vi "Curve Length Preparation.vi"(2 "formula":string) -> (0 "correct number of variables":bool, 1 "valid formula":bool, 3 "error":bool, 4 "string without spaces":string, 5 "epsilon with brackets":string, 6 "epsilon without brackets":string, 7 "formula with brackets":string)   [LabVIEW 2020, in "NI_Gmath.lvlib"]
uses:
  NI_Gmath.lvlib
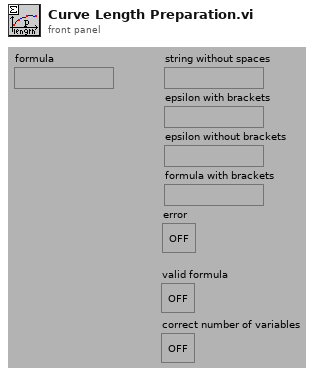
[diagram p1: front panel]
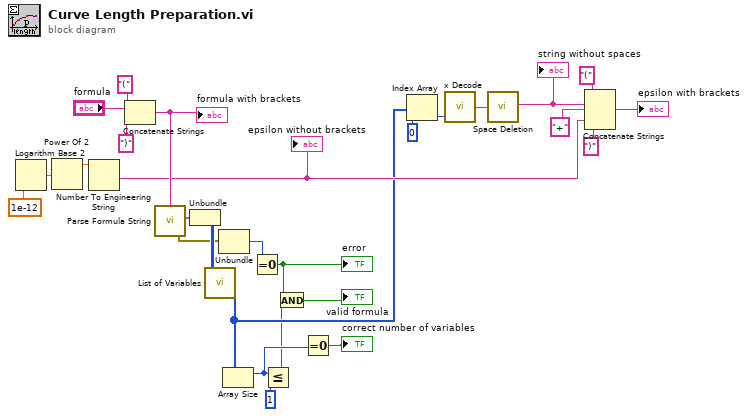
[diagram p0: block diagram]
diagram:
  n1 = Logarithm Base 2(1:1e-12) -> (0:w5:dbl)
  n2 = Power Of 2(x=w5) -> (2^x=w9:dbl)
  n3 = Number To Engineering String(4:w9) -> (0:w14:string)  [unwired: 3 in]
  "epsilon without brackets" <- w14
  n4 = Concatenate Strings("(", "formula", ")") -> (w27:string)
  "formula with brackets" <- w27
  n5 = call "Parse Formula String.vi"("formula"=w27) -> ("error out"=w15:errorcluster, "Parsed Formula"=w20:cluster{"Table":i32[][], "Y Values":dbl[]})  [unwired: 1 in]
  n6 = Unbundle(w20) -> ("Table"=w21:i32[][])  [unwired: 1 out]
  n7 = call "List of Variables.vi"("Table"=w21) -> ("List of variables"=w6:i32[])
  n8 = Unbundle(w15) -> ("code"=w16:i32)  [unwired: 2 out]
  n9 = Array Size(array=w6) -> (size(s)=w18:i32)
  n10 = Equal To 0?(x=w16) -> (x = 0?=w17:bool)
  "error" <- w17
  n11 = Less Or Equal?(x=w18, y=1) -> (x <= y?=w3:bool)
  n12 = And(x=w17, y=w3) -> (x .and. y?=→"valid formula":bool)
  n13 = Equal To 0?(x=w18) -> (x = 0?=→"correct number of variables":bool)
  n14 = Index Array(array=w6, index=0) -> (element=w8:i32)
  n15 = call "x Decode.vi"("number"=w8) -> ("x string"=w11:string)  [unwired: 1 in, 1 out]
  n16 = call "Space Deletion.vi"("string with spaces"=w11) -> ("string without spaces"=w22:string)
  "string without spaces" <- w22
  n17 = Concatenate Strings("(", w22, "+", w14, ")") -> (→"epsilon with brackets":string)
